vi "CreateTimeoutNotifier.vi"(8 "error in (no error)":errorcluster, 11 "Timeout (ms) (5000)":u32) -> (0 "error out":errorcluster, 3 "Lockin Error Timeout":refnum<notifier>)   [LabVIEW 2019, in "AFM_Litho_Plugin.IV.lvclass"]
uses:
  AFM_Litho_Plugin.IV.lvclass
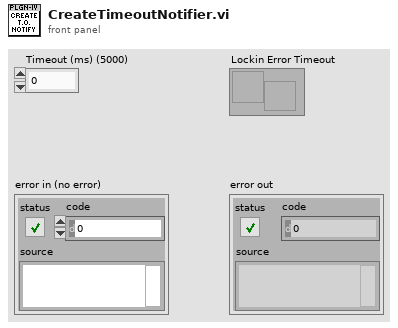
[diagram p1: front panel]
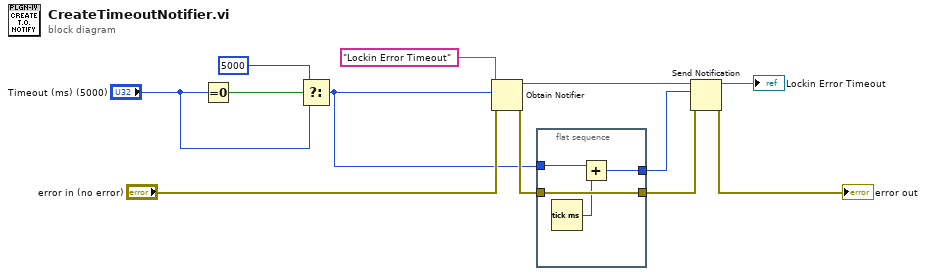
[diagram p0: block diagram]
diagram:
  n1 = Equal To 0?(x="Timeout (ms) (5000)") -> (x = 0?=w12:bool)
  n2 = Select(t=u32 5000, s=w12, f="Timeout (ms) (5000)") -> (s? t:f=w2:u32)
  n3 = Obtain Notifier(name (unnamed)="Lockin Error Timeout", notification data type=w2, error in (no error)="error in (no error)") -> (notifier out=w7:refnum<notifier>, error out=w4:errorcluster)  [unwired: 1 in, 1 out]
  n4 = flat-sequence {
    tunnel: w4 -> [w16]
    tunnel: [w16] -> w3
    tunnel: w2 -> [w14]
    tunnel: [w13] -> w1
    frame #0 {
      n5 = Tick Count (ms)() -> (millisecond timer value=w15:u32)
      n6 = Add(x=w14, y=w15) -> (x+y=w13:u32)
    }
  }
  n7 = Send Notification(notification=w1, notifier=w7, error in (no error)=w3) -> (notifier out=→"Lockin Error Timeout":refnum<notifier>, error out=→"error out":errorcluster)
